vi "Create Trigger.vi"(8 "error in (no error)":errorcluster, 11 "Async in":refnum<class "VS Inline Async API.lvclass">) -> (0 "error out":errorcluster, 3 "Async out":refnum<class "VS Inline Async API.lvclass">)   [LabVIEW 2015, in "VS Inline Async API.lvlib" / "VS Inline Async API.lvclass"]
uses:
  <vilib>/addons/Inline Async API/_VS Inline Async API/VS Inline Async API/VS Inline Async API.lvclass
  <vilib>/addons/Inline Async API/_VS Inline Async API/VS Inline Async API/VS Inline Async API.lvclass/VS Inline Async API.ctl
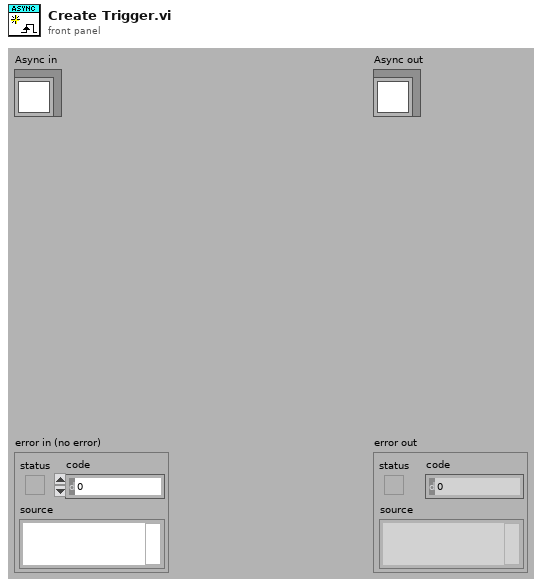
[diagram p1: front panel]
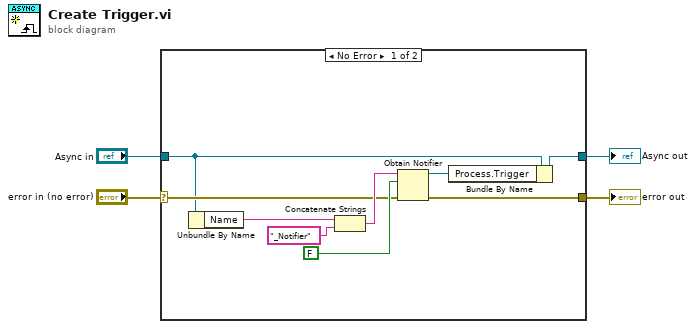
[diagram p0: block diagram]
diagram:
  n1 = case shown="No Error" "error in (no error)" {
    selector: "error in (no error)" -> [w9 w14]
    tunnel: [w13 w14] -> w4
    tunnel: "Async in" -> [w7 w15]
    tunnel: [w6 w15] -> w1
    frame No Error {
      n2 = Unbundle By Name(w7) -> ("Name"=w8:string)
      n3 = Concatenate Strings(w8, "_Notifier" ("name (unnamed)")) -> (w11:string)
      n4 = Obtain Notifier(name (unnamed)=w11, notification data type=FALSE, error in (no error)=w9) -> (notifier out=w5:refnum<notifier>, error out=w13:errorcluster)  [unwired: 1 in, 1 out]
      n5 = Bundle By Name(cluster=w7, "Process.Trigger"=w5) -> (w6:refnum<class "VS Inline Async API.lvclass">)
    }
    frame Error {
    }
  }
  "error out" <- w4
  "Async out" <- w1
